vi "PLL data source -- mfli.vi"(6 "set-get delay (msec)":i64, 7 "data source action":T1=enum."get", 9 "z  in (V)":cdb, 10 "Freq in (Hz)":dbl=40000.0 format="%#_13g") -> (1 "z out (V)":cdb=0.00010527635459-2.9308681405e-05i, 2 "Freq out (Hz)":dbl=55115.2)   [LabVIEW 2018]
uses:
  data source action.ctl
  publisher action.ctl
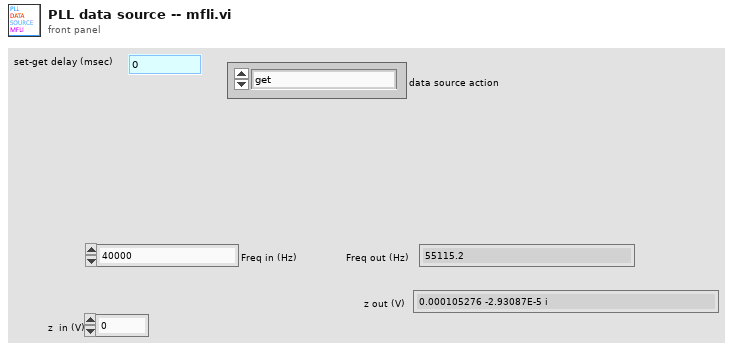
[diagram p1: front panel]
types:
  T1 = typedef "data source action.ctl" = enum16{"set", "get", "init", "set-and-get"}
  T2 = typedef "publisher action.ctl" = enum16{"set", "get", "init", "check"}
  T3 = typedef "Zurich Instruments LabOne.lvlib/ziTypeHandle.ctl" = cluster{"handleValid":bool, "Conn":u64, "Path Prefix":string, "Handle":u64, "Connected":bool, "Clockbase(s)":dbl}
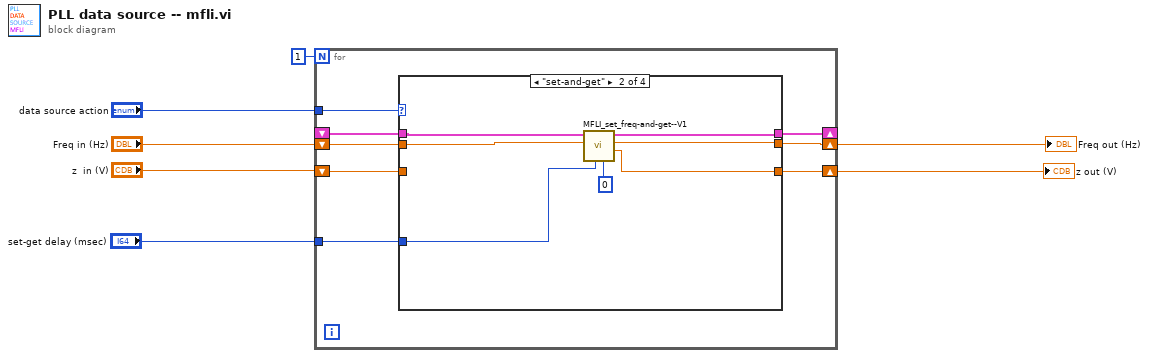
[diagram p0: block diagram]
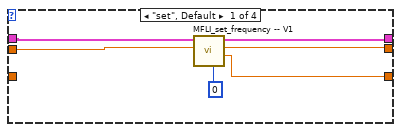
[diagram p2: hidden frame]
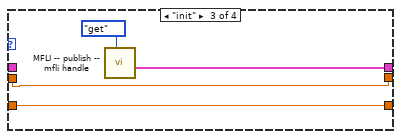
[diagram p3: hidden frame]
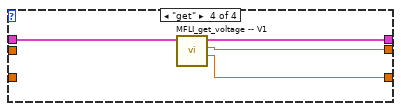
[diagram p4: hidden frame]
diagram:
  n1 = for {
    N: 1 -> [_]
    shift-right: [w15] -> _
    shift-left: _ -> [w14]
    shift-right: [w13] -> w6
    shift-left: "Freq in (Hz)" -> [w11]
    shift-right: [w12] -> w2
    shift-left: "z  in (V)" -> [w10]
    tunnel: "data source action" -> [w9]
    tunnel: "set-get delay (msec)" -> [w8]
    n2 = case shown="\"set-and-get\"" w9 {
      tunnel: [w21 w28 w31 w36] -> w15
      tunnel: w14 -> [w20 w27 _ w35]
      tunnel: [w17 w24 w29 w34] -> w13
      tunnel: [w16 w23 w30 w33] -> w12
      tunnel: w11 -> [w18 w25 w29 _]
      tunnel: w10 -> [_ _ w30 _]
      tunnel: w8 -> [_ w22 _ _]
      frame "set", Default {
        n3 = call "MFLI_set_frequency -- V1.vi"("Oscillator (0)"=u16 0, "Freq in (Hz)"=w18, "Handle In"=w20) -> ("z out (V)"=w16:cdb, "Freq out (Hz)"=w17:dbl, "Handle Out"=w21:T3)  [unwired: 5 in, 1 out]
      }
      frame "set-and-get" {
        n4 = call "MFLI_set_freq-and-get--V1.vi"("Oscillator (0)"=u16 0, "delay-circle(msec)"=w22, "Freq in (Hz)"=w25, "Handle In"=w27) -> ("z out (V)"=w23:cdb, "Freq out (Hz)"=w24:dbl, "Handle Out"=w28:T3)  [unwired: 4 in, 1 out]
      }
      frame "init" {
        n5 = call "MFLI -- publish -- mfli handle.vi"("publisher action"=publisher_action."get") -> ("Handle Out"=w31:T3)  [unwired: 10 in]
      }
      frame "get" {
        n6 = call "MFLI_get_voltage -- V1.vi"("Handle In"=w35) -> ("z out (V)"=w33:cdb, "Freq out (Hz)"=w34:dbl, "Handle Out"=w36:T3)  [unwired: 7 in, 1 out]
      }
    }
  }
  "Freq out (Hz)" <- w6
  "z out (V)" <- w2
